vi "TCPOpen.vi"(6 "timeout":i32, 8 "error in":errorcluster, 9 "port":u16, 10 "service name":string, 11 "StructIn":T1) -> (0 "error out":errorcluster, 3 "StructOut":T1)   [LabVIEW 2021, in "LibDan.lvlib"]
uses:
  LibDan.lvlib
  TerminalDef.ctl
  <vilib>/Utility/config.llb/Config Data RefNum.ctl
  <vilib>/Utility/config.llb/NI_LVConfig.lvlib
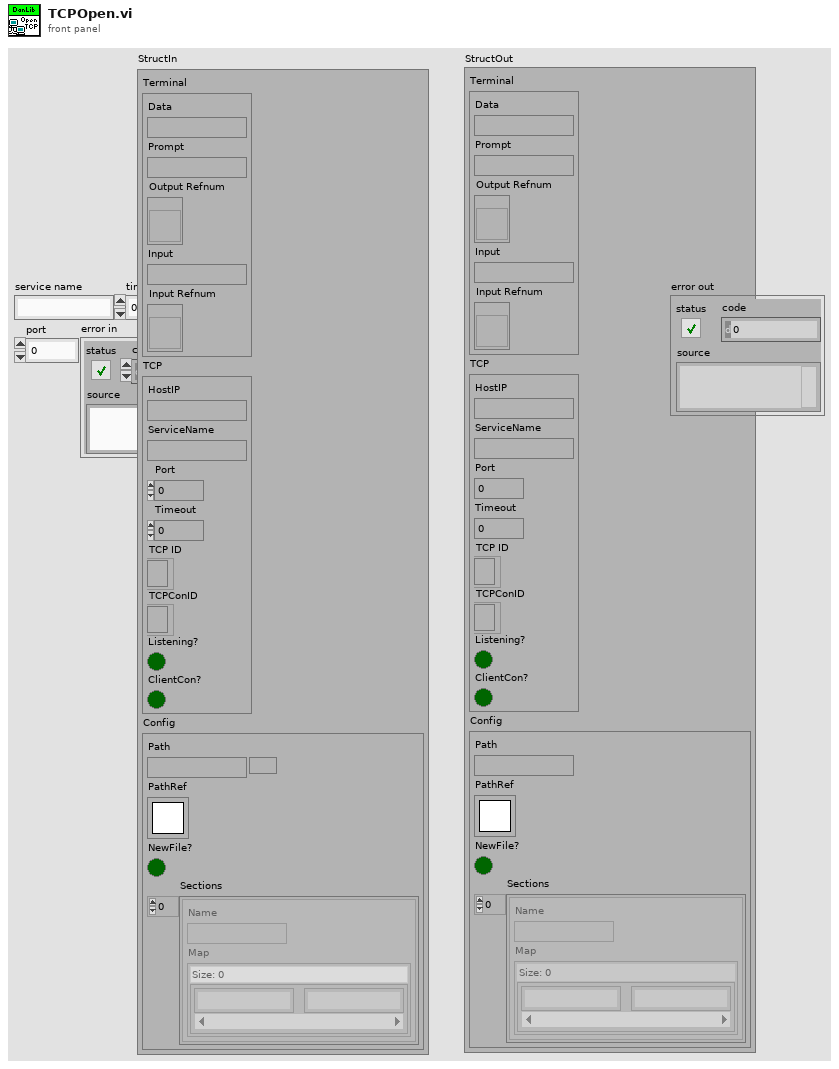
[diagram p1: front panel]
types:
  T1 = typedef "LibDan.lvlib/TerminalDef.ctl" = cluster{"Terminal":cluster{"Data":string, "Prompt":string, "Output Refnum":refnum<vi>, "Input":string, "Input Refnum":refnum<vi>}, "TCP":cluster{"HostIP":string, "ServiceName":string, "Port":u16, "Timeout":i32, "TCP ID":refnum<k5>, "TCPConID":refnum<k5>, "Listening?":bool, "ClientCon?":bool}, "Config":cluster{"Path":path, "PathRef":T2, "NewFile?":bool, "Sections":cluster{"Name":string, "Map":map{string, string}}[]}}
  T2 = typedef "NI_LVConfig.lvlib/Config Data RefNum.ctl" = refnum<k1>
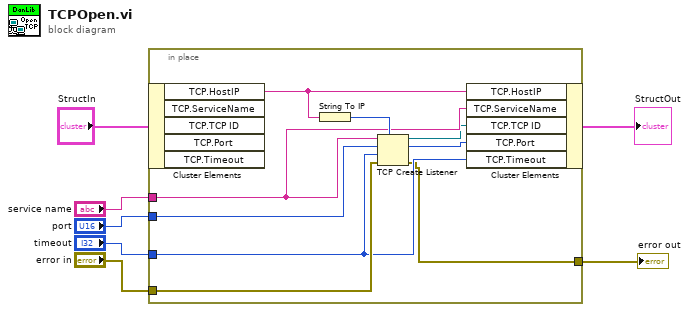
[diagram p0: block diagram]
diagram:
  n1 = in-place {
    in-place-border: "timeout" -> [w11]
    in-place-border: "error in" -> [w15]
    in-place-border: "port" -> [w14]
    in-place-border: "service name" -> [w12]
    in-place-border: [w8] -> w1
    n2 = in-place-cluster #1("StructIn") -> ("TCP.HostIP"=w13:string)  [unwired: 4 out]
    n3 = String To IP(1:w13) -> (0:w16:u32)
    n4 = TCP Create Listener(7:w16, 8:w15, 9:w11, 10:w14, 11:w12) -> (0:w8:errorcluster, 2:w9:u16, 3:w10:refnum<k5>)
    n5 = in-place-cluster #1("TCP.HostIP"=w13, "TCP.ServiceName"=w12, "TCP.TCP ID"=w10, "TCP.Port"=w9, "TCP.Timeout"=w11) -> (→"StructOut":T1)
  }
  "error out" <- w1
